vi "SetRobotProfile.vi"   [LabVIEW 2020]
doc: "Reads the robot profile from the configuration file on the roboRIO and sets any robot specific parameters."
uses:
  GlobalMiscellaneous.vi
  GlobalDrivebase.vi
  GlobalArm.vi
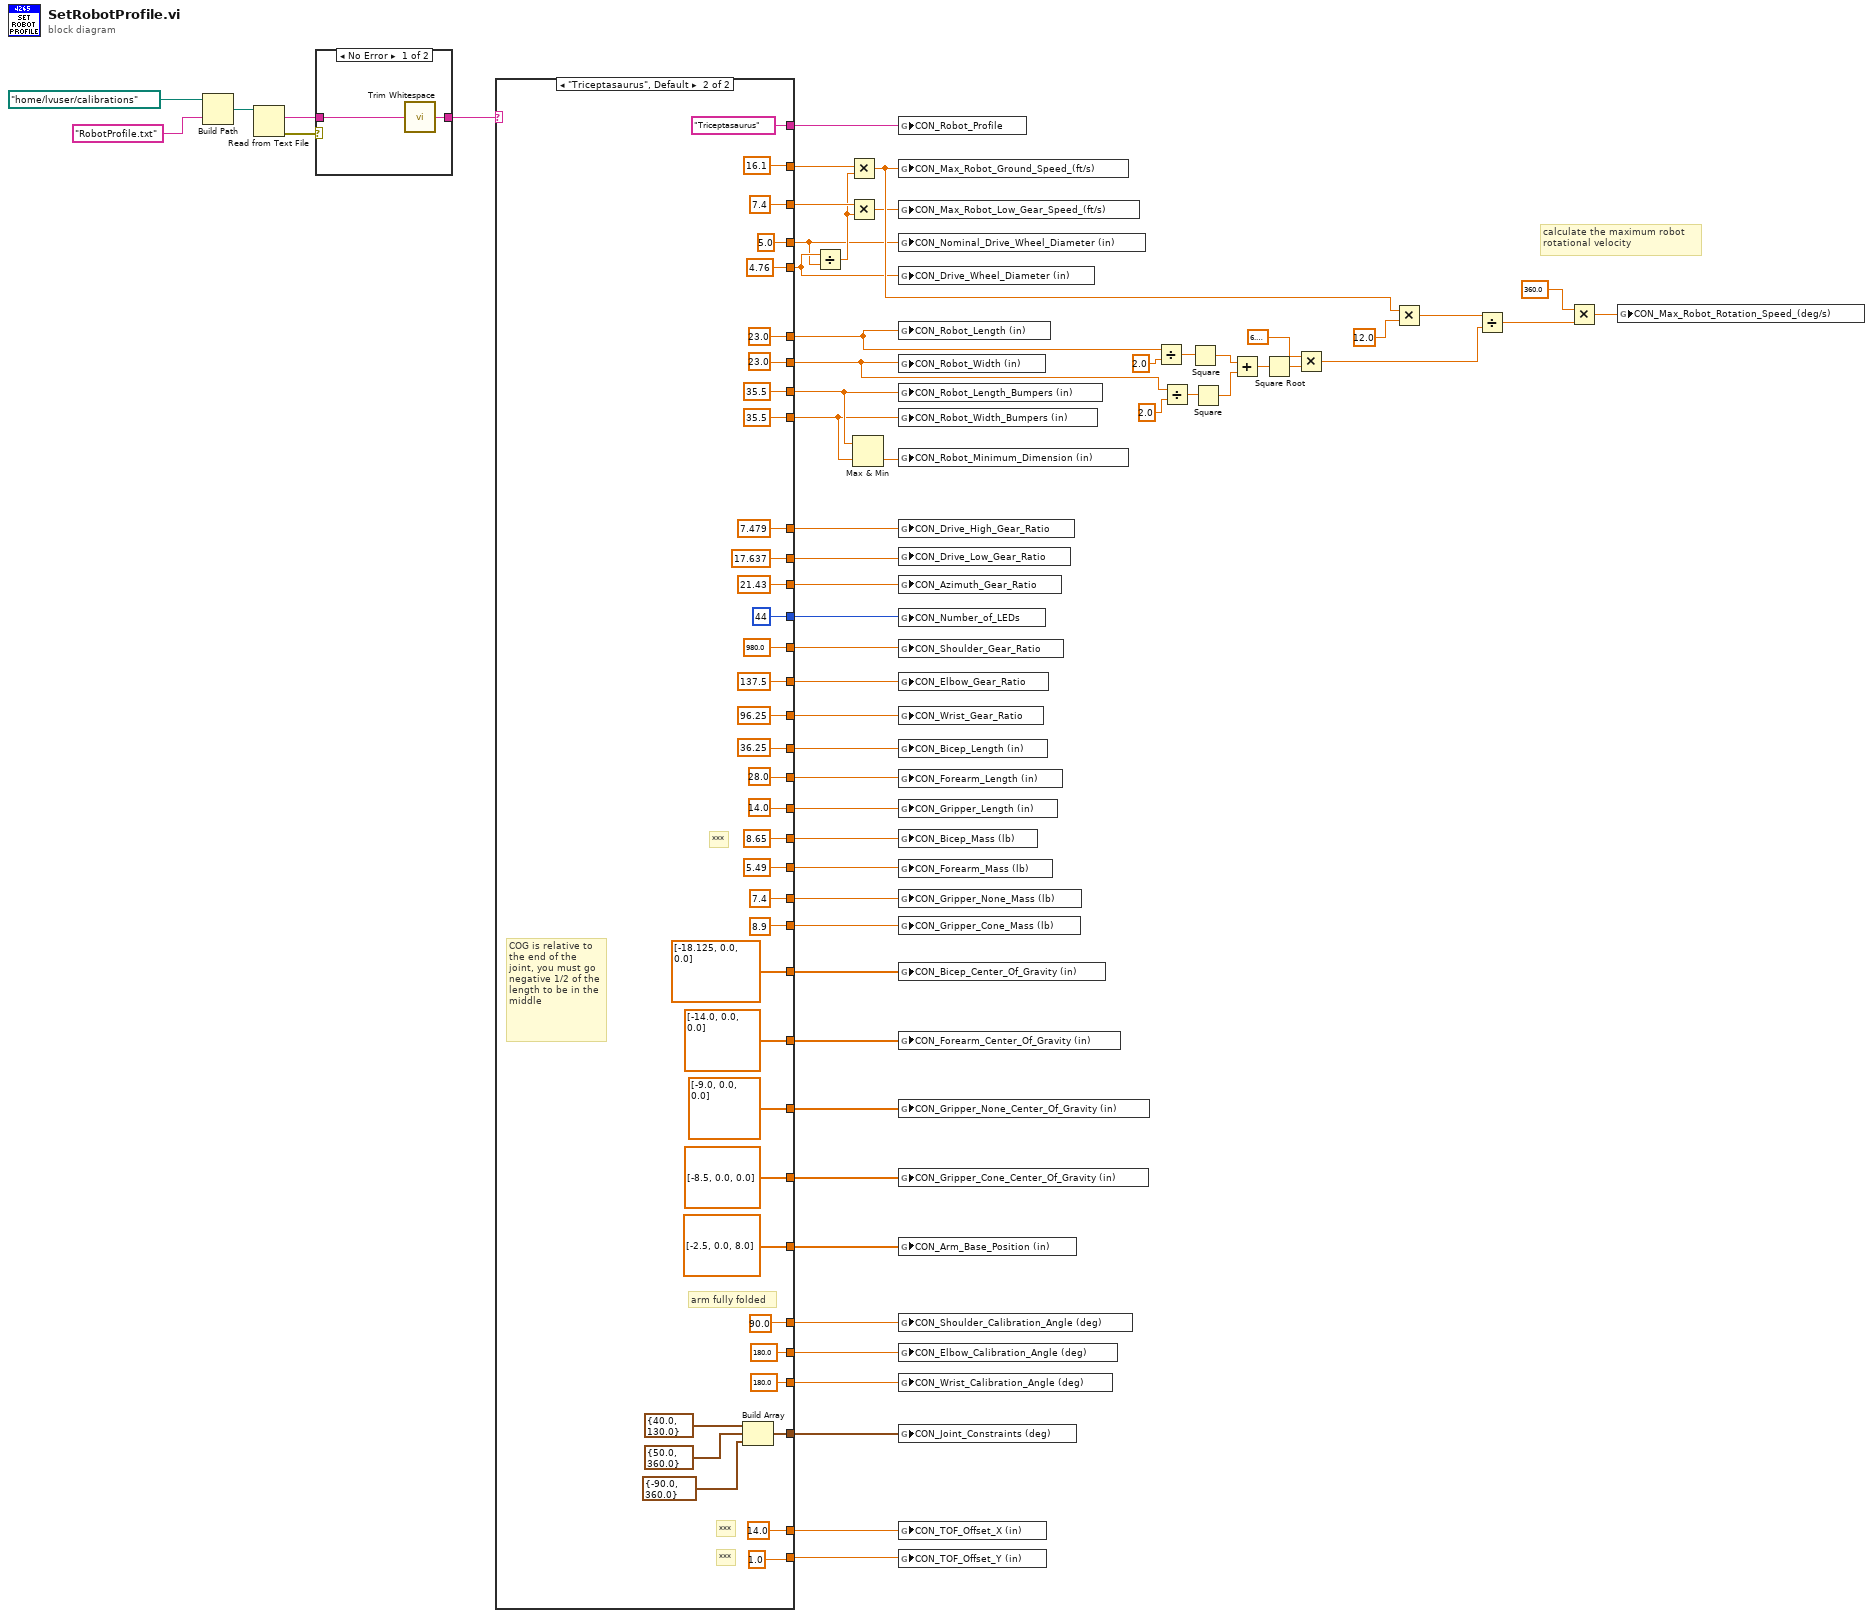
[diagram p0: block diagram]
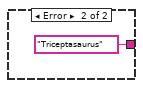
[diagram p2: hidden frame]
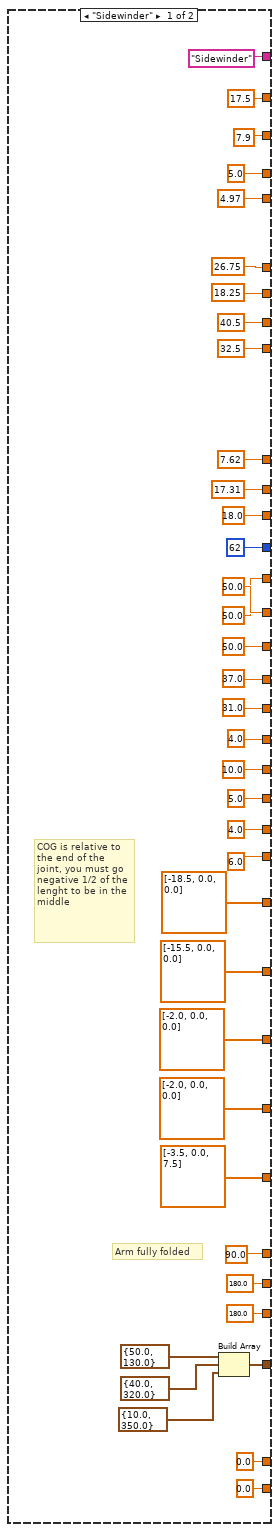
[diagram p3: hidden frame]
diagram:
  # "calculate the maximum robot\nrotational velocity"
  n1 = Build Path(base path=path "/home/lvuser/calibrations" ("path"), name or relative path="RobotProfile.txt") -> (appended path=w58:path)
  n2 = Read from Text File(file (use dialog)=w58) -> (text=w56:string, error out=w57:errorcluster)  [unwired: 3 in, 2 out]
  n3 = case shown="No Error" w57 {
    tunnel: w56 -> [w60 _]
    tunnel: [w61 "Triceptasaurus"] -> w54
    frame No Error {
      n4 = call <vilib>:"Trim Whitespace.vi"("string"=w60) -> ("trimmed string"=w61:string)  [unwired: 1 in]
    }
    frame Error {
    }
  }
  n5 = case shown="\"Triceptasaurus\", Default" w54 {
    tunnel: ["Sidewinder" "Triceptasaurus"] -> w29
    tunnel: [18.25 ("Robot_Length (in)") 23.0 ("Robot_Length (in)")] -> w38
    tunnel: [26.75 ("Robot_Length (in)") 23.0 ("Robot_Length (in)")] -> w39
    tunnel: [17.5 ("Max_Robot_Ground_Speed_(ft/s)") 16.1 ("Max_Robot_Ground_Speed_(ft/s)")] -> w9
    tunnel: [40.5 ("Robot_Length (in)") 35.5 ("Robot_Length (in)")] -> w37
    tunnel: [32.5 ("Robot_Length (in)") 35.5 ("Robot_Length (in)")] -> w36
    tunnel: [5.0 ("Robot_Length (in)") 5.0 ("Robot_Length (in)")] -> w3
    tunnel: [7.62 ("Robot_Length (in)") 7.479 ("Robot_Length (in)")] -> w34
    tunnel: [17.31 ("Robot_Length (in)") 17.637 ("Robot_Length (in)")] -> w33
    tunnel: [18.0 ("Robot_Length (in)") 21.43 ("Robot_Length (in)")] -> w32
    tunnel: [u16 62 u16 44] -> w30
    tunnel: [7.9 ("Max_Robot_Ground_Speed_(ft/s)") 7.4 ("Max_Robot_Ground_Speed_(ft/s)")] -> w7
    tunnel: [50.0 ("CON_Elbow_Gear_Ratio") 137.5 ("CON_Elbow_Gear_Ratio")] -> w28
    tunnel: [50.0 ("CON_Elbow_Gear_Ratio") 980.0 ("CON_Elbow_Gear_Ratio")] -> w27
    tunnel: [50.0 ("CON_Elbow_Gear_Ratio") 96.25 ("CON_Elbow_Gear_Ratio")] -> w26
    tunnel: [37.0 ("CON_Elbow_Gear_Ratio") 36.25 ("CON_Elbow_Gear_Ratio")] -> w25
    tunnel: [31.0 ("CON_Elbow_Gear_Ratio") 28.0 ("CON_Elbow_Gear_Ratio")] -> w24
    tunnel: [4.0 ("CON_Elbow_Gear_Ratio") 14.0 ("CON_Elbow_Gear_Ratio")] -> w23
    tunnel: [10.0 ("CON_Elbow_Gear_Ratio") 8.65 ("CON_Elbow_Gear_Ratio")] -> w22
    tunnel: [5.0 ("CON_Elbow_Gear_Ratio") 5.49 ("CON_Elbow_Gear_Ratio")] -> w21
    tunnel: [4.0 ("CON_Elbow_Gear_Ratio") 7.4 ("CON_Elbow_Gear_Ratio")] -> w20
    tunnel: [6.0 ("CON_Elbow_Gear_Ratio") 8.9 ("CON_Elbow_Gear_Ratio")] -> w19
    tunnel: [dbl[] [-18.5, 0.0, 0.0] ("CON_Bicep_Center_Of_Gravity (in)") dbl[] [-18.125, 0.0, 0.0] ("CON_Bicep_Center_Of_Gravity (in)")] -> w18
    tunnel: [dbl[] [-15.5, 0.0, 0.0] ("CON_Bicep_Center_Of_Gravity (in)") dbl[] [-14.0, 0.0, 0.0] ("CON_Bicep_Center_Of_Gravity (in)")] -> w17
    tunnel: [dbl[] [-2.0, 0.0, 0.0] ("CON_Bicep_Center_Of_Gravity (in)") dbl[] [-9.0, 0.0, 0.0] ("CON_Bicep_Center_Of_Gravity (in)")] -> w16
    tunnel: [dbl[] [-2.0, 0.0, 0.0] ("CON_Bicep_Center_Of_Gravity (in)") dbl[] [-8.5, 0.0, 0.0] ("CON_Bicep_Center_Of_Gravity (in)")] -> w15
    tunnel: [dbl[] [-3.5, 0.0, 7.5] ("CON_Bicep_Center_Of_Gravity (in)") dbl[] [-2.5, 0.0, 8.0] ("CON_Bicep_Center_Of_Gravity (in)")] -> w14
    tunnel: [90.0 90.0] -> w13
    tunnel: [180.0 180.0] -> w12
    tunnel: [180.0 180.0] -> w11
    tunnel: [w66 w103] -> w10
    tunnel: [4.97 ("Robot_Length (in)") 4.76 ("Robot_Length (in)")] -> w4
    tunnel: [0.0 14.0] -> w2
    tunnel: [0.0 1.0] -> w1
    frame "Sidewinder" {
      # "Arm fully folded"
      # "COG is relative to the end of the joint, you must go negative 1/2 of the lenght to be in the middle"
      n6 = Build Array(cluster{dbl, dbl} {50.0, 130.0}, cluster{dbl, dbl} {40.0, 320.0}, cluster{dbl, dbl} {10.0, 350.0}) -> (w66:cluster{dbl, dbl}[])
    }
    frame "Triceptasaurus", Default {
      # "***"
      # "***"
      # "***"
      # "arm fully folded"
      # "COG is relative to the end of the joint, you must go negative 1/2 of the length to be in the middle"
      n7 = Build Array(cluster{dbl, dbl} {40.0, 130.0}, cluster{dbl, dbl} {50.0, 360.0}, cluster{dbl, dbl} {-90.0, 360.0}) -> (w103:cluster{dbl, dbl}[])
    }
  }
  n8 = Divide(x=w4, y=w3) -> (x/y=w5:dbl)
  n9 = Multiply(x=w9, y=w5) -> (x*y=w8:dbl)
  n10 = Multiply(x=w7, y=w5) -> (x*y=w6:dbl)
  n11 = Max & Min(x=w37, y=w36) -> (min(x,y)=w35:dbl)  [unwired: 1 out]
  n12 = global write "GlobalMiscellaneous.vi" "CON_Robot_Profile"(w29) -> ()
  n13 = global write "GlobalDrivebase.vi" "CON_Max_Robot_Ground_Speed_(ft/s)"(w8) -> ()
  n14 = global write "GlobalDrivebase.vi" "CON_Max_Robot_Low_Gear_Speed_(ft/s)"(w6) -> ()
  n15 = global write "GlobalDrivebase.vi" "CON_Nominal_Drive_Wheel_Diameter (in)"(w3) -> ()
  n16 = global write "GlobalDrivebase.vi" "CON_Drive_Wheel_Diameter (in)"(w4) -> ()
  n17 = global write "GlobalDrivebase.vi" "CON_Robot_Length (in)"(w39) -> ()
  n18 = global write "GlobalDrivebase.vi" "CON_Robot_Width (in)"(w38) -> ()
  n19 = global write "GlobalDrivebase.vi" "CON_Robot_Length_Bumpers (in)"(w37) -> ()
  n20 = global write "GlobalDrivebase.vi" "CON_Robot_Width_Bumpers (in)"(w36) -> ()
  n21 = global write "GlobalDrivebase.vi" "CON_Robot_Minimum_Dimension (in)"(w35) -> ()
  n22 = global write "GlobalDrivebase.vi" "CON_Drive_High_Gear_Ratio"(w34) -> ()
  n23 = global write "GlobalDrivebase.vi" "CON_Drive_Low_Gear_Ratio"(w33) -> ()
  n24 = global write "GlobalDrivebase.vi" "CON_Azimuth_Gear_Ratio"(w32) -> ()
  n25 = global write "GlobalMiscellaneous.vi" "CON_Number_of_LEDs"(w30) -> ()
  n26 = global write "GlobalArm.vi" "CON_Shoulder_Gear_Ratio"(w27) -> ()
  n27 = global write "GlobalArm.vi" "CON_Elbow_Gear_Ratio"(w28) -> ()
  n28 = global write "GlobalArm.vi" "CON_Wrist_Gear_Ratio"(w26) -> ()
  n29 = global write "GlobalArm.vi" "CON_Bicep_Length (in)"(w25) -> ()
  n30 = global write "GlobalArm.vi" "CON_Forearm_Length (in)"(w24) -> ()
  n31 = global write "GlobalArm.vi" "CON_Gripper_Length (in)"(w23) -> ()
  n32 = global write "GlobalArm.vi" "CON_Bicep_Mass (lb)"(w22) -> ()
  n33 = global write "GlobalArm.vi" "CON_Forearm_Mass (lb)"(w21) -> ()
  n34 = global write "GlobalArm.vi" "CON_Gripper_None_Mass (lb)"(w20) -> ()
  n35 = global write "GlobalArm.vi" "CON_Gripper_Cone_Mass (lb)"(w19) -> ()
  n36 = global write "GlobalArm.vi" "CON_Bicep_Center_Of_Gravity (in)"(w18) -> ()
  n37 = global write "GlobalArm.vi" "CON_Forearm_Center_Of_Gravity (in)"(w17) -> ()
  n38 = global write "GlobalArm.vi" "CON_Gripper_None_Center_Of_Gravity (in)"(w16) -> ()
  n39 = global write "GlobalArm.vi" "CON_Gripper_Cone_Center_Of_Gravity (in)"(w15) -> ()
  n40 = global write "GlobalArm.vi" "CON_Arm_Base_Position (in)"(w14) -> ()
  n41 = global write "GlobalArm.vi" "CON_Shoulder_Calibration_Angle (deg)"(w13) -> ()
  n42 = global write "GlobalArm.vi" "CON_Elbow_Calibration_Angle (deg)"(w12) -> ()
  n43 = global write "GlobalArm.vi" "CON_Wrist_Calibration_Angle (deg)"(w11) -> ()
  n44 = global write "GlobalArm.vi" "CON_Joint_Constraints (deg)"(w10) -> ()
  n45 = global write "GlobalMiscellaneous.vi" "CON_TOF_Offset_X (in)"(w2) -> ()
  n46 = global write "GlobalMiscellaneous.vi" "CON_TOF_Offset_Y (in)"(w1) -> ()
  n47 = Divide(x=w39, y=2.0) -> (x/y=w45:dbl)
  n48 = Divide(x=w38, y=2.0) -> (x/y=w44:dbl)
  n49 = Square(x=w45) -> (x^2=w43:dbl)
  n50 = Square(x=w44) -> (x^2=w42:dbl)
  n51 = Add(x=w43, y=w42) -> (x+y=w41:dbl)
  n52 = Square Root(x=w41) -> (sqrt(x)=w40:dbl)
  n53 = Multiply(x=6.283185307179586, y=w40) -> (x*y=w50:dbl)
  n54 = Multiply(x=w8, y=12.0) -> (x*y=w52:dbl)
  n55 = Divide(x=w52, y=w50) -> (x/y=w49:dbl)
  n56 = Multiply(x=360.0, y=w49) -> (x*y=w31:dbl)
  n57 = global write "GlobalDrivebase.vi" "CON_Max_Robot_Rotation_Speed_(deg/s)"(w31) -> ()
